vi "Rename Document.vi"(8 "error in":errorcluster, 11 "Device In":T2) -> (0 "error out":errorcluster, 2 "Comm":T1, 3 "Device Out":T2)   [LabVIEW 2019]
uses:
  _SubVI/Cluster.ctl
  <userlib>/IoT Devices/_subVIs/HTTPComm.ctl
panel:
  in  "cancel":bool
  in  "OK Button":bool
  in  "List of files":u16(ring) items=["nameismilan", "cocacola", "pepsi", "mountain Dew", "milan", "new document", "x", "xsa", "latestdoc ", "milan", "latest doc", "milan", "something", "qq", "HELLO MILAN boss", "very cool", "HELLO MILAN", "new", "OnShape_Placemat_Glasses Challenge.pdf", "Untitled document"]
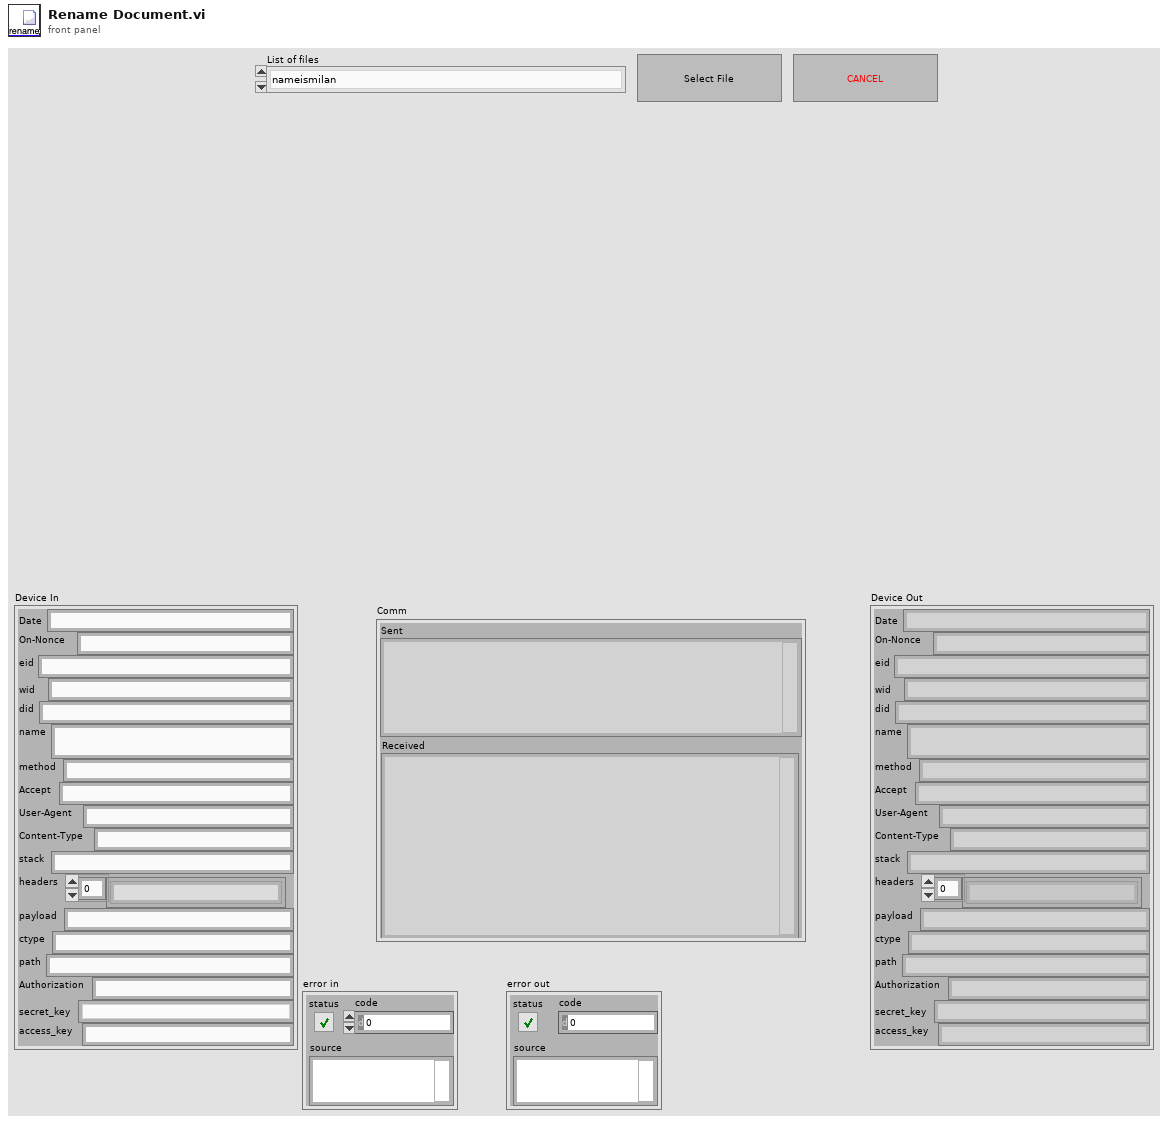
[diagram p1: front panel]
types:
  T1 = typedef "HTTPComm.ctl" = cluster{"url":string, "sent headers":string, "sent body":string, "headers":string, "body":string, "Sent":string, "Received":string}
  T2 = typedef "Cluster.ctl" = cluster{"Date":string, "On-Nonce":string, "eid":string, "wid":string, "did":string, "name":string, "method":string, "Accept":string, "User-Agent":string, "Content-Type":string, "stack":string, "headers":string[], "payload":string, "ctype":string, "path":string, "Authorization":string, "secret_key":string, "access_key":string}
  T3 = enum32{"Invalid", "Standard", "Closed", "Hidden", "Minimized", "Maximized"}
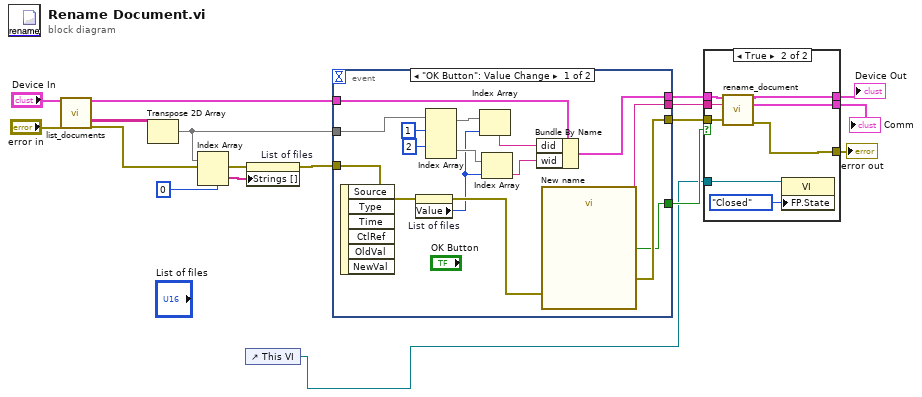
[diagram p0: block diagram]
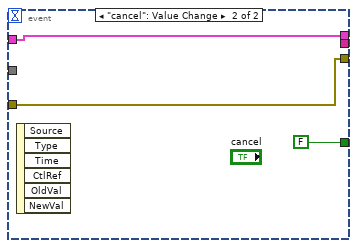
[diagram p3: hidden frame]
diagram:
  n1 = call "list_documents.vi"("Device In"="Device In", "error in"="error in") -> ("Device Out"=w17:T2, "Document list"=w16:string[][], "error out"=w13:errorcluster)  [unwired: 14 in, 1 out]
  n2 = Transpose 2D Array(2D array=w16) -> (transposed array=w11:string[][])
  n3 = Index Array(array=w11, index (row)=0) -> (element=w14:string[])  [unwired: 1 in]
  n4 = control-ref of="This VI"() -> (w1:refnum<vi>)
  n5 = property on="List of files" class="Ring (strict)"(error in=w13, "Strings []"=w14) -> (error out=w12:errorcluster)  [unwired: 1 in, 1 out]
  n6 = event shown="[0] \"OK Button\": Value Change" {
    selector: _ -> [_ _]
    dyn-events: _ -> [_ _]
    timeout: _ -> [_ _]
    tunnel: w17 -> [w32 w35]
    tunnel: w12 -> [w28 w34]
    tunnel: w11 -> [w26 _]
    tunnel: [w25 w35] -> w8
    tunnel: [w24 _] -> w7
    tunnel: [w23 w34] -> w6
    tunnel: [w22 FALSE] -> w2
    event "OK Button": Value Change {
      n7 = event-data() -> ()  [unwired: 1 in, 6 out]
      n8 = property on="List of files" class="Ring (strict)"(error in=w28) -> (error out=w27:errorcluster, "Value"=w19:u16)  [unwired: 1 in, 1 out]
      n9 = Index Array(array=w26, index (row) #1=1 ("index (row)"), index (row) #2=2 ("index (row)")) -> (element #1=w31:string[], element #2=w20:string[])  [unwired: 2 in]
      n10 = Index Array(array=w31, index=w19) -> (element=w29:string)
      n11 = Index Array(array=w20, index=w19) -> (element=w18:string)
      n12 = Bundle By Name(cluster=w32, "did"=w29, "wid"=w18) -> (w25:T2)
      n13 = call "New name"("error in (no error)"=w27) -> ("New name"=w24:string, "Change"=w22:bool, "error out"=w23:errorcluster)  [unwired: 16 in]
    }
    event "cancel": Value Change {
      n14 = event-data() -> ()  [unwired: 1 in, 6 out]
    }
  }
  n15 = case shown="True" w2 {
    tunnel: w8 -> [w37 w45]
    tunnel: w7 -> [_ w44]
    tunnel: w6 -> [w36 w43]
    tunnel: [w37 w42] -> w5
    tunnel: [w36 w41] -> w4
    tunnel: [_ w40] -> w3
    tunnel: w1 -> [_ w38]
    frame False {
    }
    frame True {
      n16 = call "rename_document.vi"("Device In"=w45, "New Name"=w44, "error in"=w43) -> ("Device Out"=w42:T2, "Comm"=w40:T1, "error out"=w41:errorcluster)  [unwired: 10 in]
      n17 = property class="VI"(reference=w38, "FP.State"=T3."Closed" ("Front Panel Window:State")) -> ()  [unwired: 1 in, 2 out]
    }
  }
  "Device Out" <- w5
  "error out" <- w4
  "Comm" <- w3
